vi "Building Current Freq response edit.vi"(6 "F variable":dbl, 7 "Vin":dbl, 8 "C":dbl, 9 "L":dbl, 10 "R":dbl, 11 "Circuit Type Enum":T1) -> (0 "Fo":dbl, 1 "Xc":dbl, 2 "Xl":dbl, 3 "Supply Current":dbl)   [LabVIEW 2019]
uses:
  Types/Circuit Type Enum.ctl
panel:
  out "Impedence":dbl
  out "IL":dbl
  out "Ic":dbl
  out "ZL":dbl
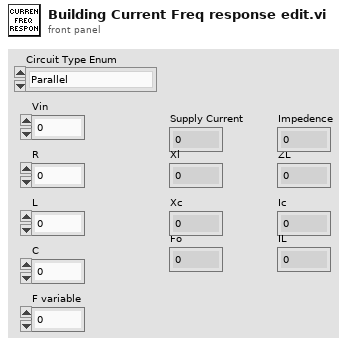
[diagram p1: front panel]
types:
  T1 = typedef "Circuit Type Enum.ctl" = enum16{"Parallel", "Serial"}
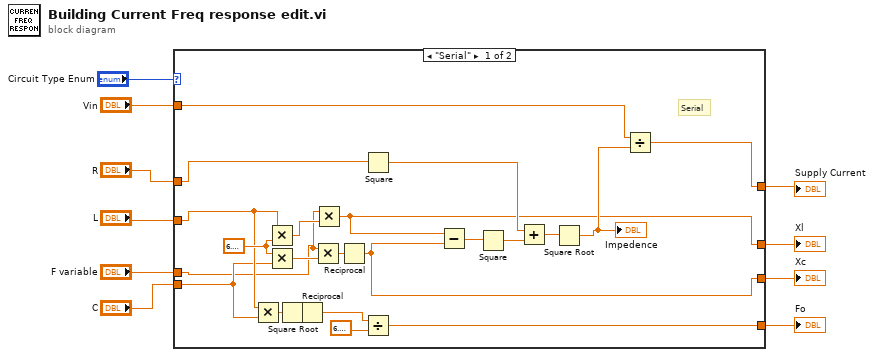
[diagram p0: block diagram]
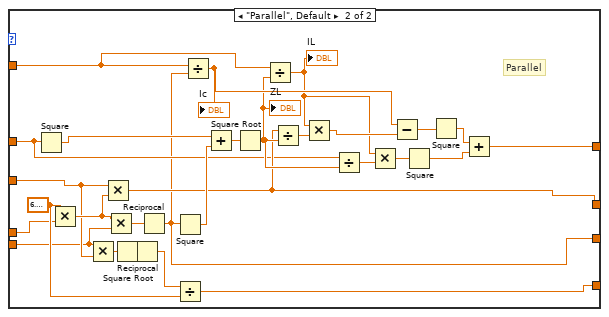
[diagram p2: hidden frame]
diagram:
  n1 = case shown="\"Serial\"" "Circuit Type Enum" {
    tunnel: [w18 w41] -> w10
    tunnel: [w11 w40] -> w4
    tunnel: "R" -> [w13 w36]
    tunnel: "F variable" -> [w14 w39]
    tunnel: "L" -> [w16 w38]
    tunnel: "Vin" -> [w17 w37]
    tunnel: [w19 w35] -> w5
    tunnel: [w12 w34] -> w3
    tunnel: "C" -> [w15 w33]
    frame "Serial" {
      w32 = 6.283185307179586
      # "Serial"
      n2 = Multiply(x=w16, y=w15) -> (x*y=w23:dbl)
      n3 = Multiply(x=w16, y=w32) -> (x*y=w31:dbl)
      n4 = Multiply(x=w32, y=w15) -> (x*y=w30:dbl)
      n5 = Square Root(x=w23) -> (sqrt(x)=w22:dbl)
      n6 = Reciprocal(x=w22) -> (1/x=w20:dbl)
      n7 = Multiply(x=w14, y=w30) -> (x*y=w29:dbl)
      n8 = Multiply(x=w14, y=w31) -> (x*y=w11:dbl)
      n9 = Reciprocal(x=w29) -> (1/x=w12:dbl)
      n10 = Square(x=w13) -> (x^2=w26:dbl)
      n11 = Divide(x=w20, y=6.283185307179586) -> (x/y=w19:dbl)
      n12 = Subtract(x=w11, y=w12) -> (x-y=w28:dbl)
      n13 = Square(x=w28) -> (x^2=w27:dbl)
      n14 = Add(x=w26, y=w27) -> (x+y=w25:dbl)
      n15 = Square Root(x=w25) -> (sqrt(x)=w24:dbl)
      "Impedence" <- w24
      n16 = Divide(x=w17, y=w24) -> (x/y=w18:dbl)
    }
    frame "Parallel", Default {
      w43 = 6.283185307179586
      # "Parallel"
      n17 = Square(x=w36) -> (x^2=w42:dbl)
      n18 = Multiply(x=w43, y=w39) -> (x*y=w60:dbl)
      n19 = Multiply(x=w33, y=w38) -> (x*y=w46:dbl)
      n20 = Multiply(x=w38, y=w60) -> (x*y=w40:dbl)
      n21 = Multiply(x=w60, y=w33) -> (x*y=w59:dbl)
      n22 = Square Root(x=w46) -> (sqrt(x)=w45:dbl)
      n23 = Reciprocal(x=w45) -> (1/x=w44:dbl)
      n24 = Reciprocal(x=w59) -> (1/x=w34:dbl)
      n25 = Square(x=w34) -> (x^2=w58:dbl)
      n26 = Divide(x=w44, y=w43) -> (x/y=w35:dbl)
      n27 = Divide(x=w37, y=w34) -> (x/y=w55:dbl)
      "Ic" <- w55
      n28 = Add(x=w42, y=w58) -> (x+y=w57:dbl)
      n29 = Square Root(x=w57) -> (sqrt(x)=w52:dbl)
      "ZL" <- w52
      n30 = Divide(x=w37, y=w52) -> (x/y=w50:dbl)
      "IL" <- w50
      n31 = Divide(x=w40, y=w52) -> (x/y=w56:dbl)
      n32 = Multiply(x=w50, y=w56) -> (x*y=w53:dbl)
      n33 = Divide(x=w36, y=w52) -> (x/y=w51:dbl)
      n34 = Multiply(x=w50, y=w51) -> (x*y=w49:dbl)
      n35 = Subtract(x=w55, y=w53) -> (x-y=w54:dbl)
      n36 = Square(x=w49) -> (x^2=w47:dbl)
      n37 = Square(x=w54) -> (x^2=w48:dbl)
      n38 = Add(x=w48, y=w47) -> (x+y=w41:dbl)
    }
  }
  "Supply Current" <- w10
  "Fo" <- w5
  "Xl" <- w4
  "Xc" <- w3
